vi "Get Log File Segmenting.vi"(8 "error in":errorcluster, 11 "log file in":T2 format="%.0x") -> (0 "error out":errorcluster, 1 "file segmenting mode":T1, 2 "segment into multiple files":bool, 3 "log file out":T2 format="%.0x", 4 "file length (s) or size (MB)":u32)   [LabVIEW 2027, in "Embedded Data Logger Scripting.lvlib"]
uses:
  Embedded Data Logger Scripting.lvlib
  <vilib>/NI VeriStand/Custom Device API/Custom Device Item Ref.ctl
  Shared/Segment Files By.ctl
  Shared/Constants.vi
  <vilib>/NI VeriStand/Custom Device API/Get Item Property (U16).vi
  <vilib>/NI VeriStand/Custom Device API/Get Item Property (U32).vi
  <vilib>/NI VeriStand/Custom Device API/Get Item Property (Boolean).vi
  <vilib>/NI VeriStand/Custom Device API/Custom Device API.lvlib
  Shared/Embedded Data Logger Shared.lvlib
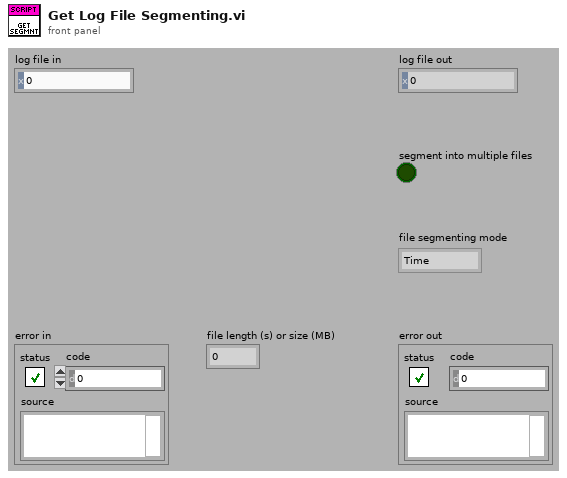
[diagram p1: front panel]
types:
  T1 = typedef "Embedded Data Logger Shared.lvlib/Segment Files By.ctl" = enum16{"Time", "Size"}
  T2 = typedef "Custom Device API.lvlib/Custom Device Item Ref.ctl" = u64
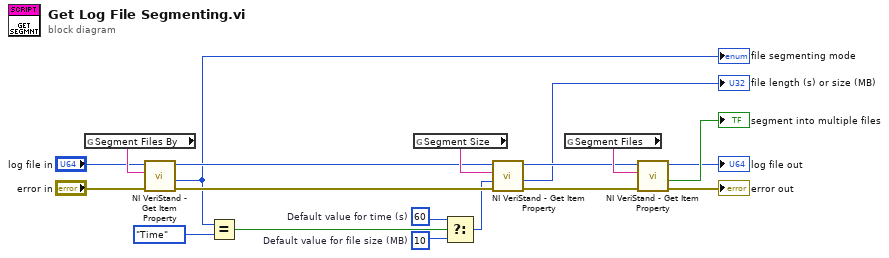
[diagram p0: block diagram]
diagram:
  w12 = u32 10  # Default value for file size (MB)
  w13 = u32 60  # Default value for time (s)
  n1 = global read "Constants.vi" "Segment Files By"() -> (w9:string)
  n2 = call-poly <vilib>:"NI VeriStand - Get Item Property.vi"("error in (no error)"="error in", "Property Name"=w9, "Item Ref in"="log file in") -> ("error out"=w5:errorcluster, "Value"=w3:u16, "Item Ref out"=w6:T2)  [unwired: 1 in, 5 out]
  "file segmenting mode" <- w3
  n3 = Equal?(x=w3, y=Segment_Files_By."Time" ("Segment Files By")) -> (x = y?=w1:bool)
  n4 = global read "Constants.vi" "Segment Size"() -> (w19:string)
  n5 = Select(t=w13, s=w1, f=w12) -> (s? t:f=w4:u32)
  n6 = call-poly <vilib>:"NI VeriStand - Get Item Property.vi"("error in (no error)"=w5, "Default Value"=w4, "Property Name"=w19, "Item Ref in"=w6) -> ("error out"=w16:errorcluster, "Value"=→"file length (s) or size (MB)":u32, "Item Ref out"=w17:T2)  [unwired: 5 out]
  n7 = global read "Constants.vi" "Segment Files"() -> (w18:string)
  n8 = call-poly <vilib>:"NI VeriStand - Get Item Property.vi"("error in (no error)"=w16, "Property Name"=w18, "Item Ref in"=w17) -> ("error out"=→"error out":errorcluster, "Value"=→"segment into multiple files":bool, "Item Ref out"=→"log file out":T2)  [unwired: 1 in, 5 out]
